vi "Load Payload.vi"(8 "error in (no error)":errorcluster, 10 "Configuration Payload":variant, 11 "CoreOOB_Rx in":refnum<class "CIFTemplateCoreOOB_Rx.lvclass">) -> (0 "error out":errorcluster, 3 "CoreOOB_Rx out":refnum<class "CIFTemplateCoreOOB_Rx.lvclass">)   [LabVIEW 2021, in "CIFTemplateCoreOOB_Rx.lvclass"]
uses:
  CIFTemplateCoreOOB_Rx.lvclass
  CIFUtilities/CIFOutOfBand/CIFOutOfBand.lvclass/CIFOutOfBand.ctl
  Typedef/Template Payload.ctl
  CIFTemplateCoreOOB_Rx.lvclass/CIFTemplateCoreOOB_Rx.ctl
  CIFUtilities/CIFOutOfBand/CIFOutOfBand.lvclass
  D:/dev/CIF-Core-LabVIEW/src/CIFUtilities/CIFOutOfBand/CIFOutOfBand.lvclass
  D:/dev/CIF-Core-LabVIEW/src/CIFTemplate/CIFTemplateCoreOOB/OOB_Rx/CIFTemplateCoreOOB_Rx.lvclass
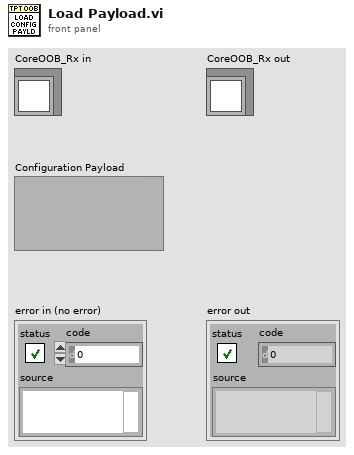
[diagram p1: front panel]
types:
  T1 = typedef "CIFTemplateCoreOOB_Rx.lvclass/Template Payload.ctl" = cluster{"Config Data":variant, "FTE":u64}
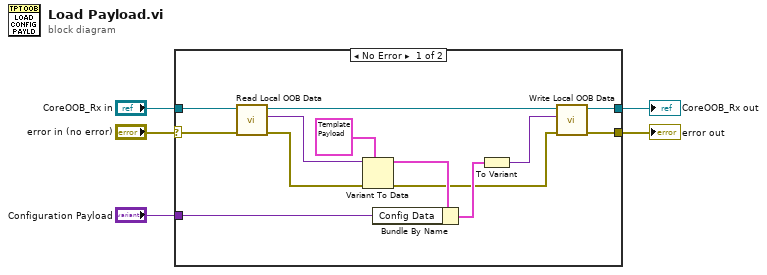
[diagram p0: block diagram]
diagram:
  n1 = case shown="No Error" "error in (no error)" {
    selector: "error in (no error)" -> [w10 w20]
    tunnel: [w18 w20] -> w5
    tunnel: [w17 w19] -> w4
    tunnel: "CoreOOB_Rx in" -> [w13 w19]
    tunnel: "Configuration Payload" -> [w16 _]
    frame No Error {
      n2 = call "Read Local OOB Data.vi"("error in"=w10, "OOB in"=w13) -> ("error out"=w7:errorcluster, "Local OOB Data"=w11:variant, "OOB out"=w12:refnum<class "CIFTemplateCoreOOB_Rx.lvclass">)  [unwired: 7 in]
      n3 = Variant To Data(error in=w7, type=T1 {"Config Data"=variant, "FTE"=0} ("Template Payload"), Variant=w11) -> (data=w8:T1, error out=w6:errorcluster)
      n4 = Bundle By Name(cluster=w8, "Config Data"=w16) -> (w15:T1)
      n5 = To Variant(anything=w15) -> (Variant=w14:variant)
      n6 = call "Write Local OOB Data.vi"("error in"=w6, "Local OOB Data"=w14, "OOB in"=w12) -> ("error out"=w18:errorcluster, "OOB out"=w17:refnum<class "CIFTemplateCoreOOB_Rx.lvclass">)  [unwired: 7 in]
    }
    frame Error {
    }
  }
  "error out" <- w5
  "CoreOOB_Rx out" <- w4
